vi "compare multiple countries window.vi"(4 "Aggregate indexes":i32[](array[numeric]), 6 "Countries":string[](array[string]), 7 "SA data":T1, 8 "US data":T1, 9 "Populations":i64[](array[numeric]), 10 "deaths CSV":string[][](array[string]), 11 "cases CSV":string[][](array[string])) -> ()   [LabVIEW 2019]
panel:
  out "population (millions)":i64
  out "Country at mouse pointer":string
  out "relative graph":cluster{"days":i32[], "Y out":dbl[]}[](graph)
  in  "include SA provinces":bool=TRUE
  in  "include aggregates":bool=TRUE
  in  "Presets":bool
  in  "include US states":bool=TRUE
  in  "Number":u16=10
  in  "Add Top countries":bool
  in  "Category":u16(ring) items=["new cases", "new deaths", "new cases per 1M", "new deaths per 1M", "rise in deaths over past 2 weeks", "fall in deaths over past 2 weeks"]
  in  "Days":u16=7 min=2
  in  "moving average":bool
  in  "Normalise Y-axis to 1M pop":bool
  in  "threshold cases":u32
  in  "Add Button":bool
  in  "Remove":bool
  in  "Countries to add":u16(ring) items=["Afghanistan", "Albania", "Algeria", "Andorra", "Angola", "Antigua and Barbuda", "Argentina", "Armenia", "Australia, Australian Capital Territory", "Australia, New South Wales", "Australia, Northern Territory", "Australia, Queensland", "Australia, South Australia", "Australia, Tasmania", "Australia, Victoria", "Australia, Western Australia", "Austria", "Azerbaijan", "Bahamas", "Bahrain", "Bangladesh", "Barbados", "Belarus", "Belgium", "Benin", "Bhutan", "Bolivia", "Bosnia and Herzegovina", "Brazil", "Brunei", "Bulgaria", "Burkina Faso", "Cabo Verde", "Cambodia", "Cameroon", "Canada, Alberta", "Canada, British Columbia", "Canada, Grand Princess", "Canada, Manitoba", "Canada, New Brunswick", "Canada, Newfoundland and Labrador", "Canada, Nova Scotia", "Canada, Ontario", "Canada, Prince Edward Island", "Canada, Quebec", "Canada, Saskatchewan", "Central African Republic", "Chad", "Chile", "China, Anhui", "China, Beijing", "China, Chongqing", "China, Fujian", "China, Gansu", "China, Guangdong", "China, Guangxi", "China, Guizhou", "China, Hainan", "China, Hebei", "China, Heilongjiang", "China, Henan", "China, Hong Kong", "China, Hubei", "China, Hunan", "China, Inner Mongolia", "China, Jiangsu", "China, Jiangxi", "China, Jilin", "China, Liaoning", "China, Macau", "China, Ningxia", "China, Qinghai", "China, Shaanxi", "China, Shandong", "China, Shanghai", "China, Shanxi", "China, Sichuan", "China, Tianjin", "China, Tibet", "China, Xinjiang", "China, Yunnan", "China, Zhejiang", "Colombia", "Congo (Brazzaville)", "Congo (Kinshasa)", "Costa Rica", "Cote d'Ivoire", "Croatia", "Diamond Princess", "Cuba", "Cyprus", "Czechia", "Denmark, Faroe Islands", "Denmark, Greenland", "Denmark", "Djibouti", "Dominican Republic", "Ecuador", "Egypt", "El Salvador", "Equatorial Guinea", "Eritrea", "Estonia", "Eswatini", "Ethiopia", "Fiji", "Finland", "France, French Guiana", "France, French Polynesia", "France, Guadeloupe", "France, Mayotte", "France, New Caledonia", "France, Reunion", "France, Saint Barthelemy", "France, St Martin", "France, Martinique", "France", "Gabon", "Gambia", "Georgia", "Germany", "Ghana", "Greece", "Guatemala", "Guinea", "Guyana", "Haiti", "Holy See", "Honduras", "Hungary", "Iceland", "India", "Indonesia", "Iran", "Iraq", "Ireland", "Israel", "Italy", "Jamaica", "Japan", "Jordan", "Kazakhstan", "Kenya", "Korea South", "Kuwait", "Kyrgyzstan", "Latvia", "Lebanon", "Liberia", "Liechtenstein", "Lithuania", "Luxembourg", "Madagascar", "Malaysia", "Maldives", "Malta", "Mauritania", "Mauritius", "Mexico", "Moldova", "Monaco", "Mongolia", "Montenegro", "Morocco", "Namibia", "Nepal", "Netherlands, Aruba", "Netherlands, Curacao", "Netherlands, Sint Maarten", "Netherlands", "New Zealand", "Nicaragua", "Niger", "Nigeria", "North Macedonia", "Norway", "Oman", "Pakistan", "Panama", "Papua New Guinea", "Paraguay", "Peru", "Philippines", "Poland", "Portugal", "Qatar", "Romania", "Russia", "Rwanda", "Saint Lucia", "Saint Vincent and the Grenadines", "San Marino", "Saudi Arabia", "Senegal", "Serbia", "Seychelles", "Singapore", "Slovakia", "Slovenia", "Somalia", "South Africa", "Spain", "Sri Lanka", "Sudan", "Suriname", "Sweden", "Switzerland", "Taiwan*", "Tanzania", "Thailand", "Togo", "Trinidad and Tobago", "Tunisia", "Turkey", "Uganda", "Ukraine", "United Arab Emirates", "United Kingdom, Bermuda", "United Kingdom, Cayman Islands", "United Kingdom, Channel Islands", "United Kingdom, Gibraltar", "United Kingdom, Isle of Man", "United Kingdom, Montserrat", "United Kingdom", "Uruguay", "US", "Uzbekistan", "Venezuela", "Vietnam", "Zambia", "Zimbabwe", "Canada, Diamond Princess", "Dominica", "Grenada", "Mozambique", "Syria", "Timor-Leste", "Belize", "Laos", "Libya", "West Bank and Gaza", "Guinea-Bissau", "Mali", "Saint Kitts and Nevis", "Canada, Northwest Territories", "Canada, Yukon", "Kosovo", "Burma", "United Kingdom, Anguilla", "United Kingdom, British Virgin Islands", "United Kingdom, Turks and Caicos Islands", "MS Zaandam", "Botswana", "Burundi", "Sierra Leone", "Netherlands, \"Bonaire Sint Eustatius and Saba\"", "Malawi", "United Kingdom, Falkland Islands (Malvinas)", "France, Saint Pierre and Miquelon", "South Sudan", "Western Sahara", "Sao Tome and Principe", "Yemen", "Comoros", "Tajikistan", "Lesotho", "Australia", "Western Europe", "Latin America", "Africa", "China", "US and Canada", "US - Northeast", "US - Midwest", "US - South", "US - West", "Scandinavia (excl Sweden)", "Middle East", "Global", "American Samoa", "Guam", "Northern Mariana Islands", "Puerto Rico", "Virgin Islands", "Alabama", "Alaska", "Arizona", "Arkansas", "California", "Colorado", "Connecticut", "Delaware", "Florida", "Georgia", "Hawaii", "Idaho", "Illinois", "Indiana", "Iowa", "Kansas", "Kentucky", "Louisiana", "Maine", "Maryland", "Massachusetts", "Michigan", "Minnesota", "Mississippi", "Missouri", "Montana", "Nebraska", "Nevada", "New Hampshire", "New Jersey", "New Mexico", "New York", "North Carolina", "North Dakota", "Ohio", "Oklahoma", "Oregon", "Pennsylvania", "Rhode Island", "South Carolina", "South Dakota", "Tennessee", "Texas", "Utah", "Vermont", "Virginia", "Washington", "West Virginia", "Wisconsin", "Wyoming"]
  in  "Data":u16(ring) items=["cumulative cases", "new cases per day", "cumulative deaths", "new deaths per day"]
  # "Select Top countries"
  # "Moving average"
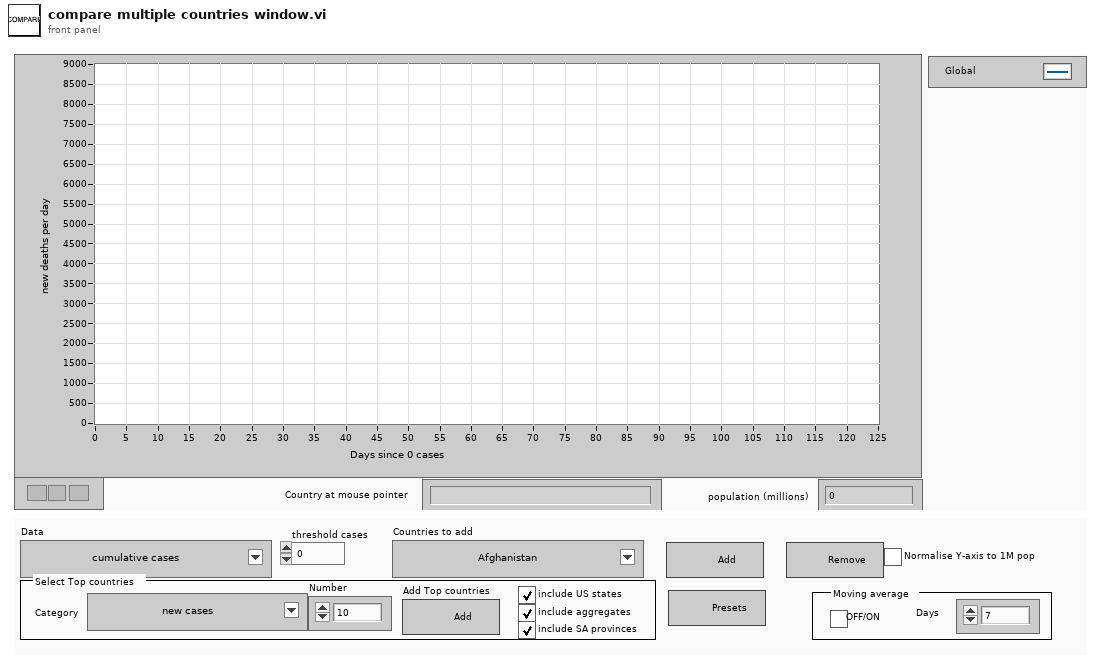
[diagram p1: front panel]
types:
  T1 = cluster{"cumulative deaths":i32[][], "deaths per day":i32[][], "case per day":i32[][], "cumulative cases":i32[][]}
  T2 = cluster{"days":i32[], "cumulative deaths":i32[]}[]
  T3 = cluster{"array index":i32[], "moving average array":dbl[]}
  T4 = cluster{"array index":i32[], "moving average array":dbl[]}[]
  T5 = cluster{"top new cases":cluster{"country index":i32[], "values":i32[]}, "top new deaths":cluster{"country index":i32[], "values":i32[]}, "top new cases per 1M":cluster{"country index":i32[], "values":dbl[]}, "top new deaths per 1M":cluster{"country index":i32[], "values":dbl[]}, "deaths dropped":cluster{"country index":i32[], "percentage change":dbl[]}, "deaths gained":cluster{"country index":i32[], "percentage change":dbl[]}, "highest deaths per day ever":cluster{"country index":i32[], "highest deaths per day":dbl[]}, "highest deaths":cluster{"country index":i32[], "highest deaths per day":dbl[]}}
  T6 = typedef "LVPoint32TypeDef.ctl" = cluster{"Horizontal":i32, "Vertical":i32}
  T7 = typedef "LVAnnotationListTypeDef.ctl" = cluster{"Name":string, "Color":u32, "Style":u8, "Point Style":u8, "Name Visible":bool, "Allow Drag":bool, "Annotation Mode":u32, "Plot":i32, "Index":i32, "Position":cluster{"X":dbl, "Y":dbl}, "X Scale":u32, "Y Scale":u32, "Show Arrow":bool, "Lock Name":bool, "Plot Area":i32, "Label Offset":cluster{"X":dbl, "Y":dbl}}[]
  T8 = cluster{"Name":string, "Color":u32, "Style":u8, "Point Style":u8, "Name Visible":bool, "Allow Drag":bool, "Annotation Mode":u32, "Plot":i32, "Index":i32, "Position":cluster{"X":dbl, "Y":dbl}, "X Scale":u32, "Y Scale":u32, "Show Arrow":bool, "Lock Name":bool, "Plot Area":i32, "Label Offset":cluster{"X":dbl, "Y":dbl}}
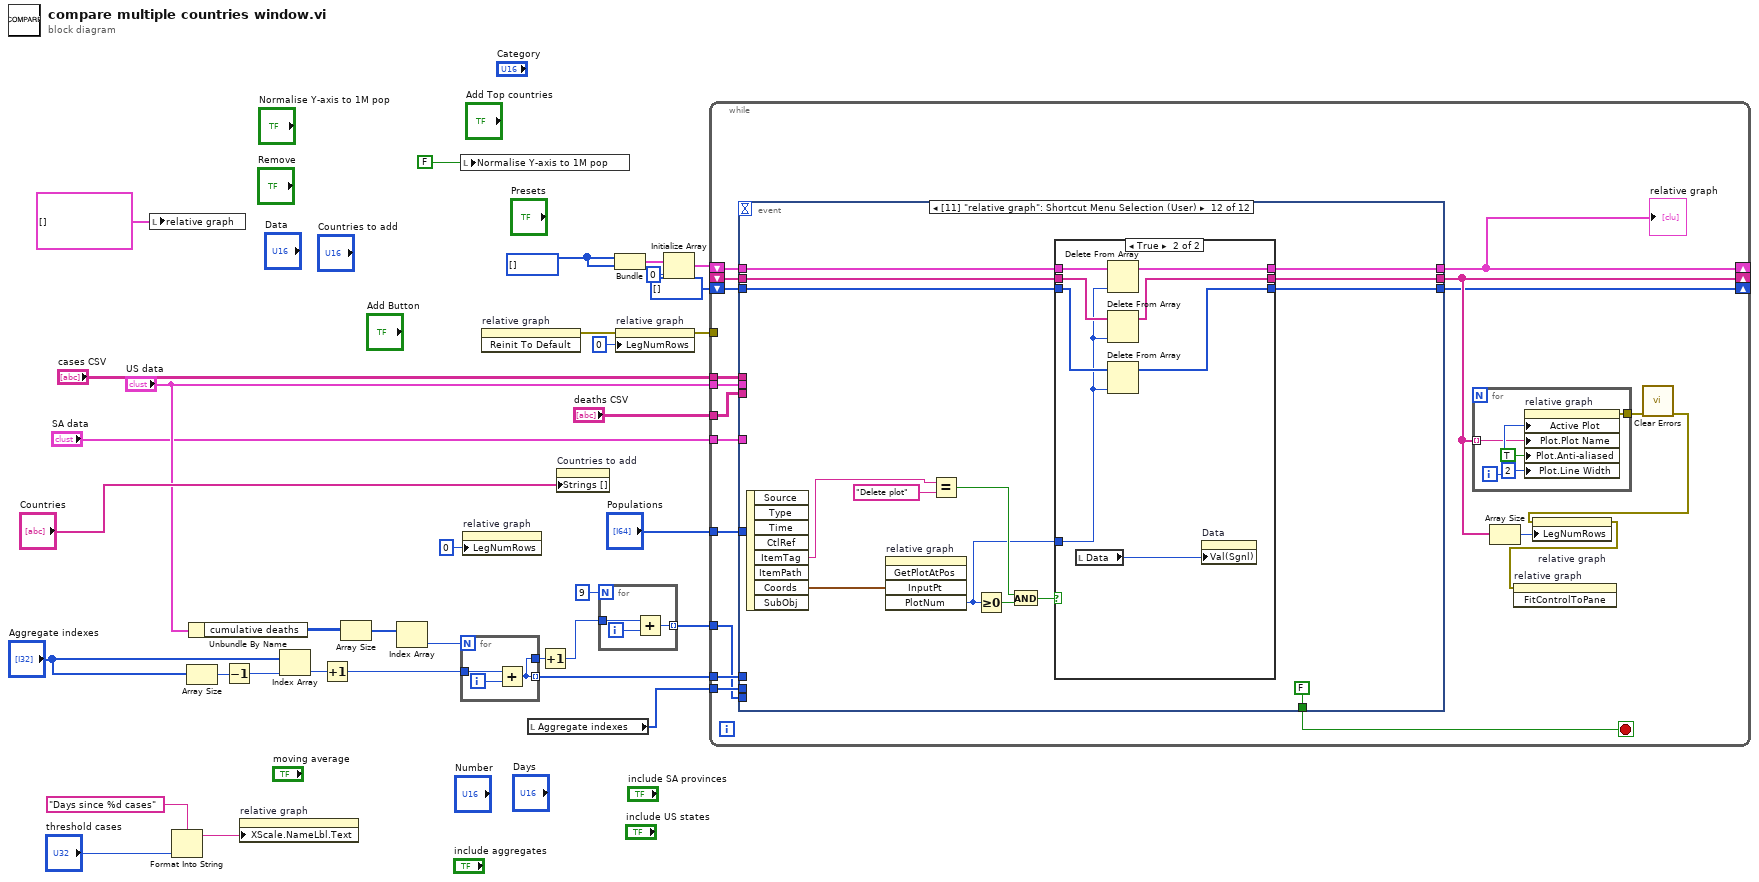
[diagram p0: block diagram]
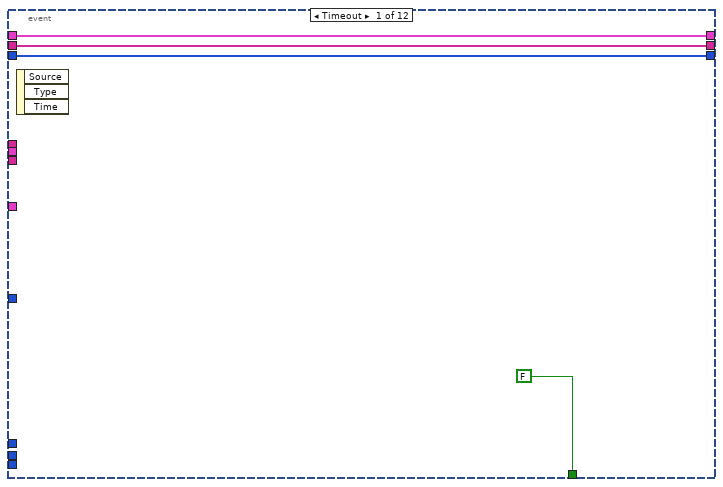
[diagram p2: hidden frame]
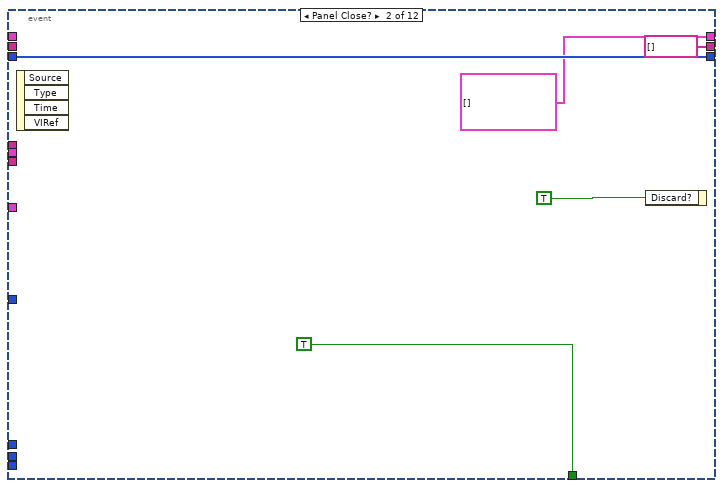
[diagram p3: hidden frame]
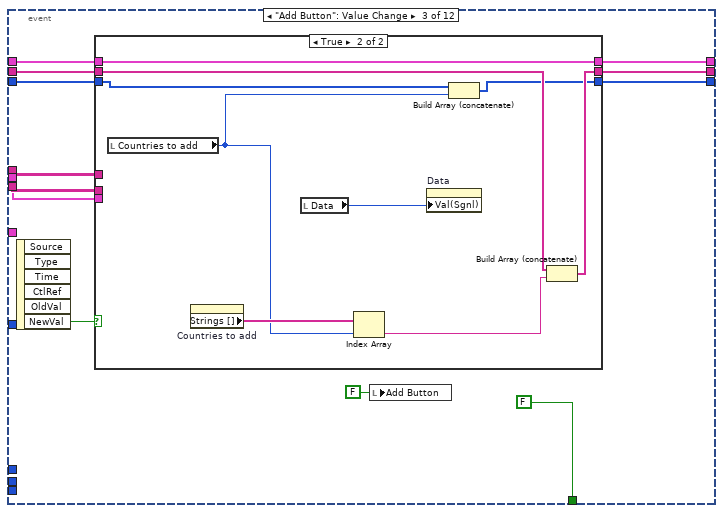
[diagram p4: hidden frame]
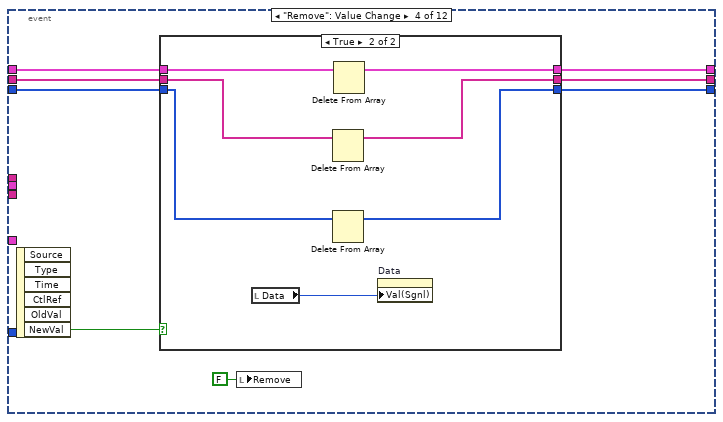
[diagram p6: hidden frame]
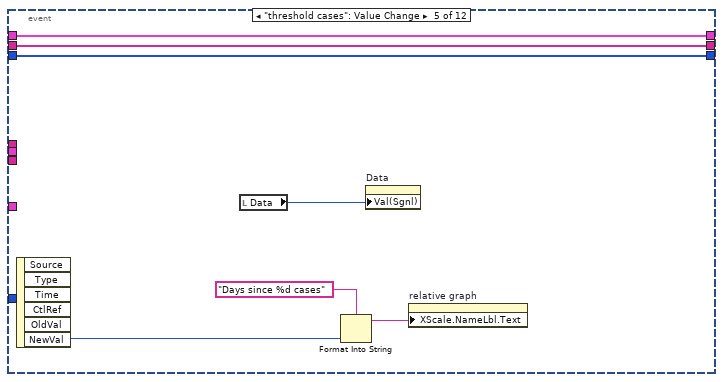
[diagram p8: hidden frame]
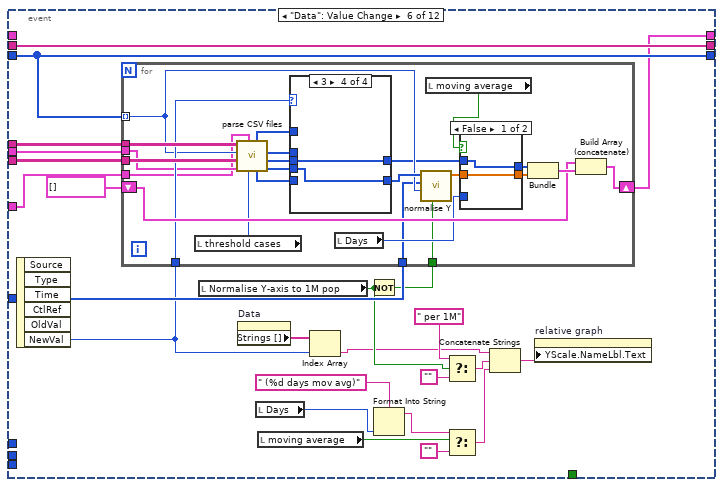
[diagram p9: hidden frame]
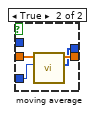
[diagram p10: hidden frame]
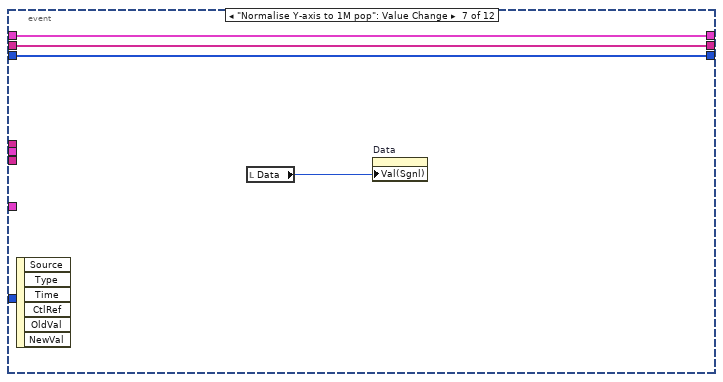
[diagram p14: hidden frame]
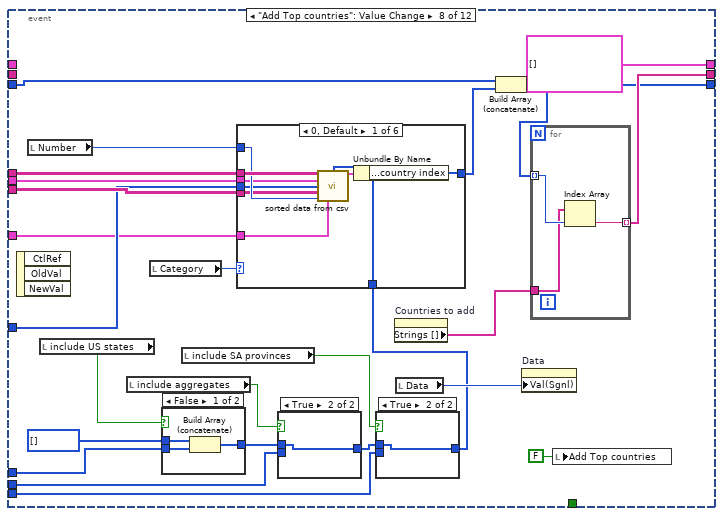
[diagram p15: hidden frame]
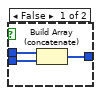
[diagram p16: hidden frame]
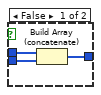
[diagram p18: hidden frame]
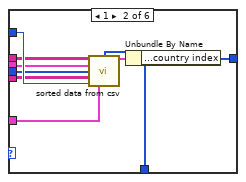
[diagram p19: hidden frame]
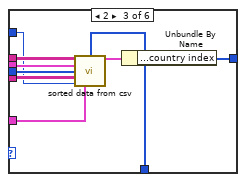
[diagram p20: hidden frame]
diagram:
  w33 = i32[] []
  n1 = local write "relative graph"(cluster{"days":i32[], "Y out":dbl[]}[] []) -> ()
  n2 = Format Into String(format string="Days since %d cases", "threshold cases") -> (resulting string=w7:string)  [unwired: 2 in, 1 out]
  n3 = Array Size(array="Aggregate indexes") -> (size(s)=w18:i32)
  n4 = Unbundle By Name("US data") -> ("cumulative deaths"=w13:i32[][])
  n5 = Decrement(x=w18) -> (x-1=w17:i32)
  n6 = property on="relative graph" class="XYGraph (strict)"("XScale.NameLbl.Text"=w7) -> ()  [unwired: 2 in, 2 out]
  n7 = Index Array(array="Aggregate indexes", index=w17) -> (element=w19:i32)
  n8 = Increment(x=w19) -> (x+1=w16:i32)
  n9 = Array Size(array=w13) -> (size(s)=w12:i32[])
  n10 = Index Array(array=w12) -> (element=w11:i32)  [unwired: 1 in]
  n11 = local write "Normalise Y-axis to 1M pop"(FALSE ("Normalise Y-axis to 1M pop")) -> ()
  n12 = for {
    N: w11 -> [_]
    tunnel: [w35] -> w10 mode=indexing
    tunnel: w16 -> [w36]
    tunnel: [w35] -> w3
    i -> [w37]
    n13 = Add(x=w36, y=w37) -> (x+y=w35:i32)
  }
  n14 = property on="relative graph" class="XYGraph (strict)"("LegNumRows"=u32 0 ("Legend:Number of Rows")) -> ()  [unwired: 2 in, 2 out]
  n15 = invoke on="relative graph" class="XYGraph (strict)" method="Reinit To Default"() -> (error out=w20:errorcluster)  [unwired: 3 in, 2 out]
  n16 = local read "Aggregate indexes"() -> (w9:i32[])
  n17 = Increment(x=w3) -> (x+1=w2:i32)
  n18 = property on="Countries to add" class="Ring (strict)"("Strings []"="Countries") -> ()  [unwired: 2 in, 2 out]
  n19 = for {
    N: 9 -> [_]
    tunnel: [w40] -> w1 mode=indexing
    tunnel: w2 -> [w38]
    i -> [w39]
    n20 = Add(x=w38, y=w39) -> (x+y=w40:i32)
  }
  n21 = Bundle(w33, w33) -> (w30:cluster{i32[], i32[]})  [unwired: 1 in]
  n22 = property on="relative graph" class="XYGraph (strict)"(error in=w20, "LegNumRows"=u32 0 ("Legend:Number of Rows")) -> (error out=w22:errorcluster)  [unwired: 1 in, 1 out]
  n23 = Initialize Array(w30, 0 ("dimension size")) -> (w32:cluster{i32[], i32[]}[])
  n24 = while {
    tunnel: "cases CSV" -> [w59]
    tunnel: "deaths CSV" -> [w58]
    shift-right: [w45] -> _
    shift-left: w32 -> [w57]
    shift-right: [w54] -> _
    shift-left: _ -> [w55]
    shift-right: [w52] -> _
    shift-left: u16[] [] -> [w51]
    tunnel: "Populations" -> [w50]
    tunnel: "US data" -> [w46]
    tunnel: w22 -> [_]
    tunnel: w10 -> [w44]
    tunnel: w9 -> [w43]
    tunnel: "SA data" -> [w42]
    tunnel: w1 -> [w41]
    stop <- w56 stop-if-true
    n25 = event shown="[11] \"relative graph\": Shortcut Menu Selection (User)" {
      selector: _ -> [_ _ _ _ _ _ _ _ _ _ _ _]
      dyn-events: _ -> [_ _ _ _ _ _ _ _ _ _ _ _]
      timeout: _ -> [_ _ _ _ _ _ _ _ _ _ _ _]
      tunnel: w59 -> [_ _ w85 _ _ w144 _ w203 _ _ _ _]
      tunnel: w58 -> [_ _ w84 _ _ w143 _ w202 _ _ _ _]
      tunnel: [w68 cluster{"days":i32[], "Y out":dbl[]}[] [] w83 w104 w120 w142 w185 cluster{"days":i32[], "Y out":dbl[]}[] [] w297 w325 w332 w361] -> w45
      tunnel: w57 -> [w68 _ w82 w105 w120 _ w185 _ w297 w325 w333 w362]
      tunnel: [FALSE TRUE FALSE _ _ _ _ _ _ _ _ FALSE] -> w56
      tunnel: [w67 string[] [] w79 w102 w122 w146 w188 w209 w296 w324 w330 w359] -> w54
      tunnel: w55 -> [w67 _ w78 w103 w122 w146 w188 _ w296 w324 w331 w360]
      tunnel: [w66 w71 w76 w98 w121 w145 w187 w207 w286 w323 w328 w357] -> w52
      tunnel: w51 -> [w66 w71 w75 w99 w121 w145 w187 w208 w286 w323 w329 w358]
      tunnel: w50 -> [_ _ _ _ _ w140 _ w200 w285 _ _ _]
      tunnel: w46 -> [_ _ w74 _ _ w137 _ w201 _ _ _ _]
      tunnel: w44 -> [_ _ _ _ _ _ _ w196 _ _ _ _]
      tunnel: w43 -> [_ _ _ _ _ _ _ w194 _ _ _ _]
      tunnel: w42 -> [_ _ _ _ _ w123 _ w189 _ _ _ _]
      tunnel: w41 -> [_ _ _ _ _ _ _ w191 _ _ _ _]
      event Timeout {
        n26 = event-data() -> ()  [unwired: 1 in, 3 out]
      }
      event Panel Close? {
        n27 = event-data() -> ()  [unwired: 1 in, 4 out]
        n28 = event-data("Discard?"=TRUE) -> ()  [unwired: 1 in, 1 out]
      }
      event "Add Button": Value Change {
        n29 = event-data() -> ("NewVal"=w81:bool)  [unwired: 1 in, 5 out]
        n30 = case shown="True" w81 {
          tunnel: w85 -> [_ _]
          tunnel: w84 -> [_ _]
          tunnel: [w88 w90] -> w83
          tunnel: w82 -> [w88 w90]
          tunnel: [w87 w95] -> w79
          tunnel: w78 -> [w87 w94]
          tunnel: [w86 w93] -> w76
          tunnel: w75 -> [w86 w92]
          tunnel: w74 -> [_ _]
          frame False {
          }
          frame True {
            n31 = local read "Countries to add"() -> (w91:u16)
            n32 = property on="Countries to add" class="Ring (strict)"() -> ("Strings []"=w97:string[])  [unwired: 2 in, 2 out]
            n33 = local read "Data"() -> (w89:u16)
            n34 = Index Array(array=w97, index=w91) -> (element=w96:string)
            n35 = property on="Data" class="Ring (strict)"("Val(Sgnl)"=w89) -> ()  [unwired: 2 in, 2 out]
            n36 = Build Array (concatenate)(w92, w91) -> (w93:i32[])
            n37 = Build Array (concatenate)(w94, w96) -> (w95:string[])
          }
        }
        n38 = local write "Add Button"(FALSE ("Add Button")) -> ()
      }
      event "Remove": Value Change {
        n39 = event-data() -> ("NewVal"=w101:bool)  [unwired: 1 in, 5 out]
        n40 = case shown="True" w101 {
          tunnel: w105 -> [w108 w115]
          tunnel: [w108 w114] -> w104
          tunnel: w103 -> [w107 w113]
          tunnel: [w107 w112] -> w102
          tunnel: w99 -> [w106 w111]
          tunnel: [w106 w110] -> w98
          frame False {
          }
          frame True {
            n41 = local read "Data"() -> (w109:u16)
            n42 = Delete From Array(array=w113) -> (array with subset deleted=w112:string[])  [unwired: 2 in, 1 out]
            n43 = Delete From Array(array=w111) -> (array with subset deleted=w110:i32[])  [unwired: 2 in, 1 out]
            n44 = Delete From Array(array=w115) -> (array with subset deleted=w114:cluster{"days":i32[], "Y out":dbl[]}[])  [unwired: 2 in, 1 out]
            n45 = property on="Data" class="Ring (strict)"("Val(Sgnl)"=w109) -> ()  [unwired: 2 in, 2 out]
          }
        }
        n46 = local write "Remove"(FALSE ("Remove")) -> ()
      }
      event "threshold cases": Value Change {
        n47 = event-data() -> ("NewVal"=w116:u32)  [unwired: 1 in, 5 out]
        n48 = local read "Data"() -> (w119:u16)
        n49 = Format Into String(format string="Days since %d cases", w116) -> (resulting string=w118:string)  [unwired: 2 in, 1 out]
        n50 = property on="Data" class="Ring (strict)"("Val(Sgnl)"=w119) -> ()  [unwired: 2 in, 2 out]
        n51 = property on="relative graph" class="XYGraph (strict)"("XScale.NameLbl.Text"=w118) -> ()  [unwired: 2 in, 2 out]
      }
      event "Data": Value Change {
        n52 = event-data() -> ("NewVal"=w138:u16)  [unwired: 1 in, 5 out]
        n53 = local read "Normalise Y-axis to 1M pop"() -> (w133:bool)
        n54 = property on="Data" class="Ring (strict)"() -> ("Strings []"=w139:string[])  [unwired: 2 in, 2 out]
        n55 = local read "Days"() -> (w124:u16)
        n56 = local read "moving average"() -> (w128:bool)
        n57 = Index Array(array=w139, index=w138) -> (element=w127:string)
        n58 = Not(x=w133) -> (.not. x?=w135:bool)
        n59 = for {
          tunnel: w145 -> [w157] mode=indexing
          tunnel: w144 -> [w166]
          tunnel: w143 -> [w165]
          shift-right: [w163] -> w142
          shift-left: T2 [] -> [w162]
          tunnel: w138 -> [w161]
          tunnel: w140 -> [w148]
          tunnel: w137 -> [w156]
          tunnel: w135 -> [w149]
          tunnel: w123 -> [w147]
          n60 = local read "threshold cases"() -> (w160:u32)
          n61 = call "parse CSV files.vi"("threshold cases"=w160, "SA data"=w147, "US data"=w156, "deaths CSV"=w165, "country index"=w157, "cases CSV"=w166) -> ("new deaths per day"=w159:i32[], "days"=w169:i32[], "new cases per day"=w168:i32[], "cumulative cases"=w170:i32[], "cumulative deaths"=w167:i32[])  [unwired: 1 out]
          n62 = case shown="3" w161 {
            tunnel: w170 -> [w177 _ _ _]
            tunnel: w169 -> [w178 w180 w182 w184]
            tunnel: [w178 w180 w182 w184] -> w152
            tunnel: [w177 w179 w181 w183] -> w158
            tunnel: w168 -> [_ w179 _ _]
            tunnel: w167 -> [_ _ w181 _]
            tunnel: w159 -> [_ _ _ w183]
            frame 0, Default {
            }
            frame 1 {
            }
            frame 2 {
            }
            frame 3 {
            }
          }
          n63 = local read "Days"() -> (w153:u16)
          n64 = call "normalise Y.vi"("Y-axis absolute"=w149, "Country index"=w157, "Populations"=w148, "Y in"=w158) -> ("Y out"=w155:dbl[])  [unwired: 7 in]
          n65 = local read "moving average"() -> (w150:bool)
          n66 = case shown="False" w150 {
            tunnel: w155 -> [w171 w176]
            tunnel: [w171 w175] -> w154
            tunnel: w153 -> [_ w174]
            tunnel: w152 -> [w172 _]
            tunnel: [w172 w173] -> w151
            frame False {
            }
            frame True {
              n67 = call "moving average.vi"("average over x points"=w174, "Array"=w176) -> ("array index"=w173:i32[], "moving average array"=w175:dbl[])  [unwired: 8 in]
            }
          }
          n68 = Bundle("array index"=w151, "moving average array"=w154) -> (w164:T3)  [unwired: 1 in]
          n69 = Build Array (concatenate)(w162, w164) -> (w163:T4)
        }
        n70 = Format Into String(format string=" (%d days mov avg)", w124) -> (resulting string=w126:string)  [unwired: 2 in, 1 out]
        n71 = Select(t=" per 1M", s=w133, f="") -> (s? t:f=w134:string)
        n72 = Select(t=w126, s=w128, f="") -> (s? t:f=w130:string)
        n73 = Concatenate Strings(w127, w134, w130) -> (w136:string)
        n74 = property on="relative graph" class="XYGraph (strict)"("YScale.NameLbl.Text"=w136) -> ()  [unwired: 2 in, 2 out]
      }
      event "Normalise Y-axis to 1M pop": Value Change {
        n75 = event-data() -> ()  [unwired: 1 in, 6 out]
        n76 = local read "Data"() -> (w186:u16)
        n77 = property on="Data" class="Ring (strict)"("Val(Sgnl)"=w186) -> ()  [unwired: 2 in, 2 out]
      }
      event "Add Top countries": Value Change {
        n78 = event-data() -> ()  [unwired: 1 in, 3 out]
        n79 = local read "Number"() -> (w204:u16)
        n80 = local read "include US states"() -> (w197:bool)
        n81 = local read "include aggregates"() -> (w199:bool)
        n82 = local read "Category"() -> (w212:u16)
        n83 = case shown="False" w197 {
          tunnel: w196 -> [w220 _]
          tunnel: [w219 w221] -> w195
          tunnel: i32[] [] ("Aggregate indexes") -> [w218 w221]
          frame False {
            n84 = Build Array (concatenate)(w218, w220) -> (w219:i32[])
          }
          frame True {
          }
        }
        n85 = local read "include SA provinces"() -> (w193:bool)
        n86 = case shown="True" w199 {
          tunnel: w194 -> [w224 _]
          tunnel: [w223 w225] -> w192
          tunnel: w195 -> [w222 w225]
          frame False {
            n87 = Build Array (concatenate)(w222, w224) -> (w223:i32[])
          }
          frame True {
          }
        }
        n88 = case shown="True" w193 {
          tunnel: w191 -> [w216 _]
          tunnel: [w215 w217] -> w190
          tunnel: w192 -> [w214 w217]
          frame False {
            n89 = Build Array (concatenate)(w214, w216) -> (w215:i32[])
          }
          frame True {
          }
        }
        n90 = case shown="0, Default" w212 {
          tunnel: [w230 w239 w248 w257 w273 w283] -> w211
          tunnel: w204 -> [w236 w246 w251 w260 w272 w282]
          tunnel: w203 -> [w237 w245 w255 w264 w271 w281]
          tunnel: w202 -> [w233 w244 w252 w261 w268 w278]
          tunnel: w201 -> [w235 w243 w254 w263 w270 w280]
          tunnel: w200 -> [w234 w242 w253 w262 w269 w279]
          tunnel: w190 -> [w232 w241 w250 w259 w267 w277]
          tunnel: w189 -> [w229 w238 w247 w256 w265 w275]
          frame 0, Default {
            n91 = call "sorted data from csv.vi"("cases CSV"=w237, "filter out"=w232, "US data"=w235, "Populations"=w234, "deaths CSV"=w233, "top selection"=w236, "SA data"=w229) -> ("ranked results"=w231:T5)  [unwired: 8 in]
            n92 = Unbundle By Name(w231) -> ("top new cases.country index"=w230:i32[])
          }
          frame 1 {
            n93 = call "sorted data from csv.vi"("cases CSV"=w245, "filter out"=w241, "US data"=w243, "Populations"=w242, "deaths CSV"=w244, "top selection"=w246, "SA data"=w238) -> ("ranked results"=w240:T5)  [unwired: 8 in]
            n94 = Unbundle By Name(w240) -> ("top new deaths.country index"=w239:i32[])
          }
          frame 2 {
            n95 = call "sorted data from csv.vi"("cases CSV"=w255, "filter out"=w250, "US data"=w254, "Populations"=w253, "deaths CSV"=w252, "top selection"=w251, "SA data"=w247) -> ("ranked results"=w249:T5)  [unwired: 8 in]
            n96 = Unbundle By Name(w249) -> ("top new cases per 1M.country index"=w248:i32[])
          }
          frame 3 {
            n97 = call "sorted data from csv.vi"("cases CSV"=w264, "filter out"=w259, "US data"=w263, "Populations"=w262, "deaths CSV"=w261, "top selection"=w260, "SA data"=w256) -> ("ranked results"=w258:T5)  [unwired: 8 in]
            n98 = Unbundle By Name(w258) -> ("top new deaths per 1M.country index"=w257:i32[])
          }
          frame 4 {
            n99 = call "sorted data from csv.vi"("cases CSV"=w271, "filter out"=w267, "US data"=w270, "Populations"=w269, "deaths CSV"=w268, "top selection"=w272, "SA data"=w265, "period in days to check"=14) -> ("ranked results"=w274:T5)  [unwired: 7 in]
            n100 = Unbundle By Name(w274) -> ("deaths gained.country index"=w273:i32[])
          }
          frame 5 {
            n101 = call "sorted data from csv.vi"("cases CSV"=w281, "filter out"=w277, "US data"=w280, "Populations"=w279, "deaths CSV"=w278, "top selection"=w282, "SA data"=w275, "period in days to check"=14) -> ("ranked results"=w284:T5)  [unwired: 7 in]
            n102 = Unbundle By Name(w284) -> ("deaths dropped.country index"=w283:i32[])
          }
        }
        n103 = property on="Countries to add" class="Ring (strict)"() -> ("Strings []"=w210:string[])  [unwired: 2 in, 2 out]
        n104 = local read "Data"() -> (w205:u16)
        n105 = Build Array (concatenate)(w208, w211) -> (w207:i32[])
        n106 = property on="Data" class="Ring (strict)"("Val(Sgnl)"=w205) -> ()  [unwired: 2 in, 2 out]
        n107 = for {
          tunnel: w207 -> [w228] mode=indexing
          tunnel: w210 -> [w227]
          tunnel: [w226] -> w209 mode=indexing
          n108 = Index Array(array=w227, index=w228) -> (element=w226:string)
        }
        n109 = local write "Add Top countries"(FALSE ("Add Top countries")) -> ()
      }
      event "relative graph": Mouse Move {
        n110 = event-data() -> ("Coords"=w290:T6)  [unwired: 1 in, 4 out]
        n111 = invoke on="relative graph" class="XYGraph (strict)" method="GetPlotAtPos"("InputPt"=w290) -> (error out=w295:errorcluster, "PlotNum"=w294:i32)  [unwired: 4 in, 3 out]
        n112 = invoke on="relative graph" class="XYGraph (strict)" method="Map Coords To XY"("Coords"=w290) -> ("XY"=w289:cluster{"X":dbl, "Y":dbl})  [unwired: 6 in, 6 out]
        n113 = property on="relative graph" class="XYGraph (strict)"() -> ("AnntList"=w292:T7)  [unwired: 2 in, 2 out]
        n114 = Greater Or Equal To 0?(x=w294) -> (x >= 0?=w293:bool)
        n115 = case shown="True" w293 {
          tunnel: w295 -> [_ w321]
          tunnel: w294 -> [_ w309]
          tunnel: w292 -> [w302 w315]
          tunnel: [w300 w314] -> w291
          tunnel: w289 -> [_ w311]
          tunnel: ["" ("Plot.Plot Name") w310] -> w288
          tunnel: [0 w303] -> w287
          tunnel: w286 -> [_ w308]
          tunnel: w285 -> [_ w307]
          frame False {
            n116 = Reshape Array(w302, 0 ("dimension size")) -> (w300:T7)
          }
          frame True {
            n117 = Unbundle By Name(w311) -> ("X"=w313:dbl)
            n118 = property on="relative graph" class="XYGraph (strict)"(error in=w321, "Active Plot"=w309) -> (error out=w320:errorcluster)  [unwired: 1 in, 1 out]
            n119 = Index Array(array=w308, index=w309) -> (element=w306:i32)
            n120 = Index Array(array=w307, index=w306) -> (element=w305:i64)
            n121 = property on="relative graph" class="XYGraph (strict)"(error in=w320) -> ("Plot.Plot Name"=w310:string)  [unwired: 1 in, 2 out]
            n122 = Index Array(array=w315) -> (element=w318:T8)  [unwired: 1 in]
            n123 = Bundle By Name(cluster=w318, "Name"=w310, "Position"=w311, "Allow Drag"=TRUE, "Index"=w313, "Annotation Mode"=u32 0, "Color"=u32 0) -> (w319:T8)
            n124 = Quotient & Remainder(x=w305, y=1000000) -> (floor(x/y)=w303:i64)  [unwired: 1 out]
            n125 = Replace Array Subset(array=w315, new element=w319) -> (w314:T7)  [unwired: 1 in]
          }
        }
        "Country at mouse pointer" <- w288
        "population (millions)" <- w287
        n126 = property on="relative graph" class="XYGraph (strict)"("AnntList"=w291) -> ()  [unwired: 2 in, 2 out]
      }
      event "moving average", "Days": Value Change {
        n127 = event-data() -> ()  [unwired: 1 in, 6 out]
        n128 = local read "Data"() -> (w322:u16)
        n129 = property on="Data" class="Ring (strict)"("Val(Sgnl)"=w322) -> ()  [unwired: 2 in, 2 out]
      }
      event "Presets": Value Change {
        n130 = event-data() -> ("NewVal"=w327:bool)  [unwired: 1 in, 5 out]
        n131 = case shown="True" w327 {
          tunnel: w333 -> [w336 w340]
          tunnel: [w336 w339] -> w332
          tunnel: w331 -> [w335 w338]
          tunnel: [w335 w337] -> w330
          tunnel: w329 -> [w334 w341]
          tunnel: [w334 w342] -> w328
          frame False {
          }
          frame True {
            n132 = call "presets2 dialog.vi"("Countries in"=w341) -> ("Load?"=w344:bool, "Countries out"=w343:i32[])  [unwired: 9 in]
            n133 = case shown="False" w344 {
              tunnel: w343 -> [_ w350]
              tunnel: [w347 w350] -> w342
              tunnel: w341 -> [w347 _]
              tunnel: w340 -> [w346 _]
              tunnel: [w346 cluster{"days":i32[], "Y out":dbl[]}[] []] -> w339
              tunnel: w338 -> [w345 _]
              tunnel: [w345 w348] -> w337
              frame False {
              }
              frame True {
                n134 = property on="Countries to add" class="Ring (strict)"() -> ("Strings []"=w349:string[])  [unwired: 2 in, 2 out]
                n135 = property on="Data" class="Ring (strict)"("Val(Sgnl)"=u16 3 ("Value (Signaling)")) -> ()  [unwired: 2 in, 2 out]
                n136 = for {
                  tunnel: w350 -> [w355] mode=indexing
                  tunnel: w349 -> [w354]
                  tunnel: [w353] -> w348 mode=indexing
                  n137 = Index Array(array=w354, index=w355) -> (element=w353:string)
                }
              }
            }
          }
        }
        n138 = local write "Presets"(FALSE ("Presets")) -> ()
      }
      event "relative graph": Shortcut Menu Selection (User) {
        n139 = event-data() -> ("ItemTag"=w367:string, "Coords"=w368:T6)  [unwired: 1 in, 6 out]
        n140 = invoke on="relative graph" class="XYGraph (strict)" method="GetPlotAtPos"("InputPt"=w368) -> ("PlotNum"=w356:i32)  [unwired: 4 in, 4 out]
        n141 = Equal?(x=w367, y="Delete plot") -> (x = y?=w363:bool)
        n142 = Greater Or Equal To 0?(x=w356) -> (x >= 0?=w364:bool)
        n143 = And(x=w363, y=w364) -> (x .and. y?=w365:bool)
        n144 = case shown="True" w365 {
          tunnel: w362 -> [w372 w379]
          tunnel: [w372 w378] -> w361
          tunnel: [w371 w375] -> w359
          tunnel: w360 -> [w371 w377]
          tunnel: w358 -> [w370 w376]
          tunnel: [w370 w374] -> w357
          tunnel: w356 -> [_ w373]
          frame False {
          }
          frame True {
            n145 = local read "Data"() -> (w380:u16)
            n146 = Delete From Array(array=w379, index=w373) -> (array with subset deleted=w378:cluster{"days":i32[], "Y out":dbl[]}[])  [unwired: 1 in, 1 out]
            n147 = Delete From Array(array=w377, index=w373) -> (array with subset deleted=w375:string[])  [unwired: 1 in, 1 out]
            n148 = Delete From Array(array=w376, index=w373) -> (array with subset deleted=w374:i32[])  [unwired: 1 in, 1 out]
            n149 = property on="Data" class="Ring (strict)"("Val(Sgnl)"=w380) -> ()  [unwired: 2 in, 2 out]
          }
        }
      }
    }
    "relative graph" <- w45
    n150 = for {
      tunnel: w54 -> [w63] mode=indexing
      tunnel: [w60] -> w48
      i -> [w64]
      n151 = property on="relative graph" class="XYGraph (strict)"("Active Plot"=w64, "Plot.Plot Name"=w63, "Plot.Anti-aliased"=TRUE, "Plot.Line Width"=u8 2) -> (error out=w60:errorcluster)  [unwired: 2 in, 1 out]
    }
    n152 = Array Size(array=w54) -> (size(s)=w53:i32)
    n153 = call <vilib>:"Clear Errors.vi"("error in (no error)"=w48) -> ("error out"=w47:errorcluster)  [unwired: 5 in, 1 out]
    n154 = property on="relative graph" class="XYGraph (strict)"(error in=w47, "LegNumRows"=w53) -> (error out=w49:errorcluster)  [unwired: 1 in, 1 out]
    n155 = invoke on="relative graph" class="XYGraph (strict)" method="FitControlToPane"(error in=w49) -> ()  [unwired: 2 in, 3 out]
  }
